vi "test Prepare Aliases for Editor.vi"(8 "error in (no error)":errorcluster, 11 "TestCase in":refnum<class "Routing and Faulting Unit Tests.lvclass">) -> (0 "error out":errorcluster, 3 "TestCase out":refnum<class "Routing and Faulting Unit Tests.lvclass">)   [LabVIEW 2020, in "Routing and Faulting Unit Tests.lvclass"]
uses:
  Routing and Faulting Unit Tests.lvclass
  Shared/Alias Mapping.ctl
  Shared/Alias Endpoint.ctl
  System Explorer/Alias Map by Module.ctl
  System Explorer/Possible Connections.ctl
  Shared/Routing and Faulting Hardware API/Types/Possible Connections for Endpoint.ctl
  <vilib>/addons/_JKI Toolkits/VI Tester/TestCase.llb/TestCase.lvclass
  System Explorer/Routing and Faulting System Explorer.lvlib
  Shared/Routing and Faulting Shared.lvlib
  Shared/Routing and Faulting Hardware API/Routing and Faulting Hardware API.lvlib
  C:/Program Files (x86)/National Instruments/LabVIEW 2020/vi.lib/addons/_JKI Toolkits/VI Tester/TestCase.llb/TestCase.lvclass
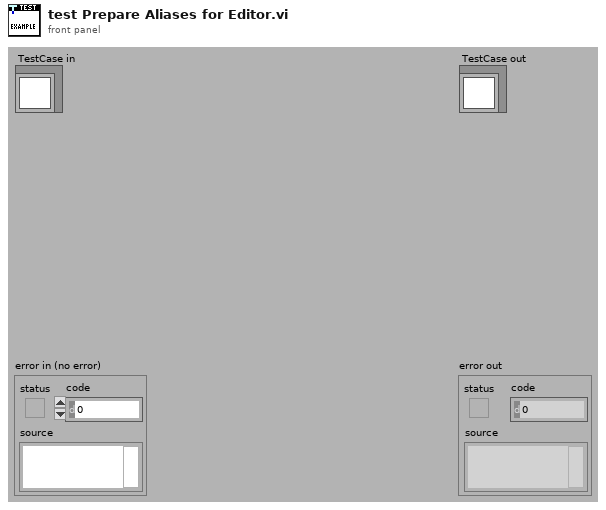
[diagram p1: front panel]
types:
  T1 = typedef "Routing and Faulting System Explorer.lvlib/Possible Connections.ctl" = cluster{" Module Path":string, "Short Module Path":string, "Product Name":string, "Possible Connections":T2[], "Missing":bool}
  T2 = typedef "Routing and Faulting Hardware API.lvlib/Possible Connections for Endpoint.ctl" = cluster{"Source":string, "Destinations":string[]}
  T3 = typedef "Routing and Faulting System Explorer.lvlib/Alias Map by Module.ctl" = cluster{"Module":string, "Alias Map":cluster{"Aliases":string[], "Endpoints":string[]}}
  T4 = typedef "Routing and Faulting Shared.lvlib/Alias Mapping.ctl" = cluster{"Alias":string, "Endpoint":T5}
  T5 = typedef "Routing and Faulting Shared.lvlib/Alias Endpoint.ctl" = cluster{"Module Path":string, "Endpoint":string}
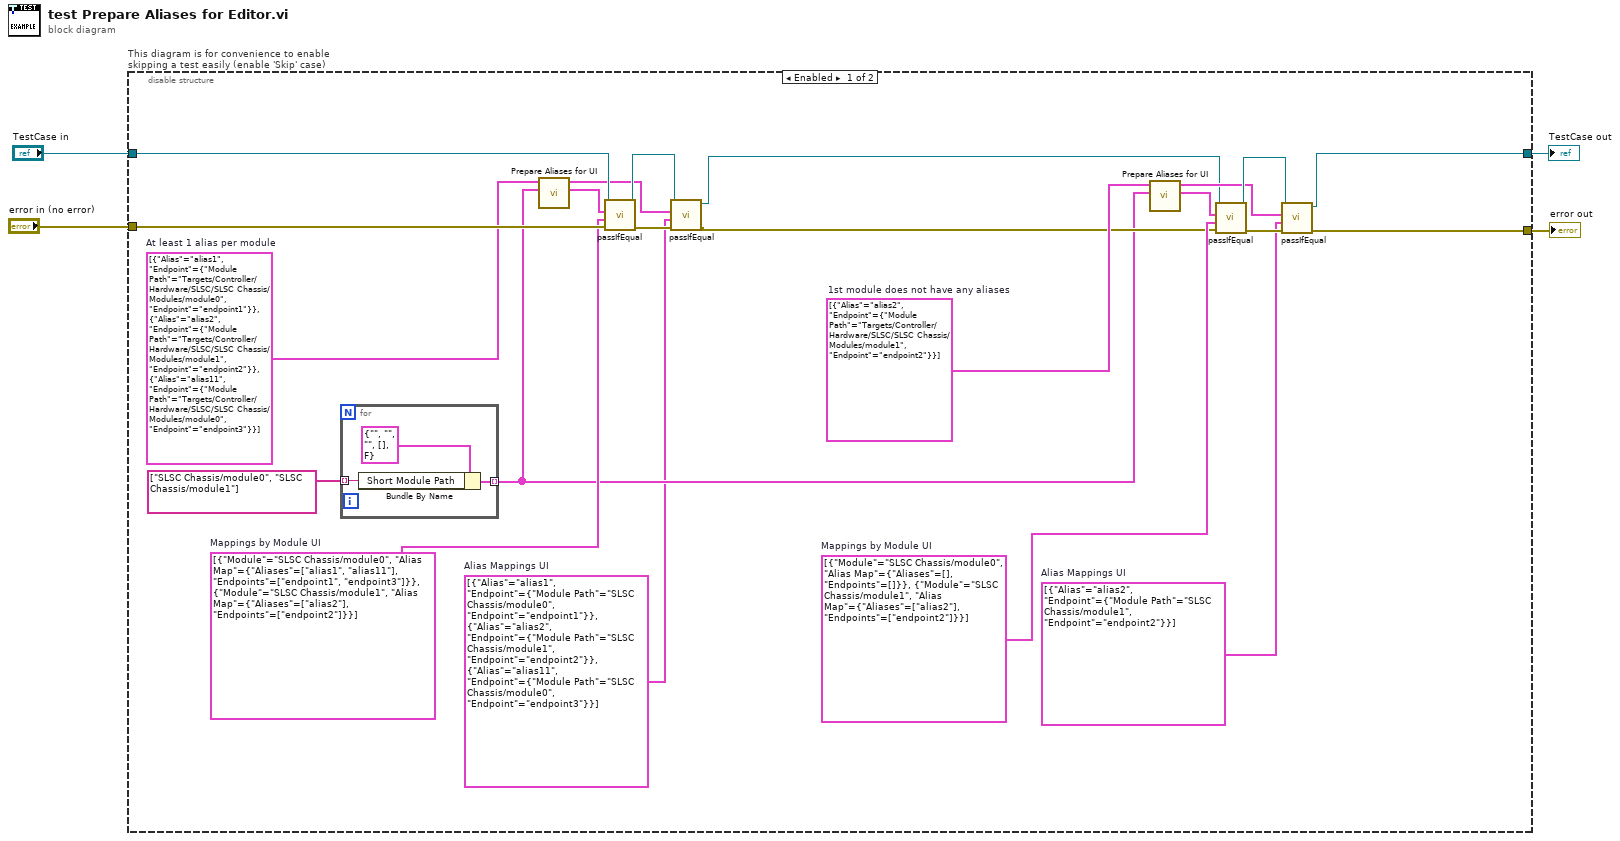
[diagram p0: block diagram]
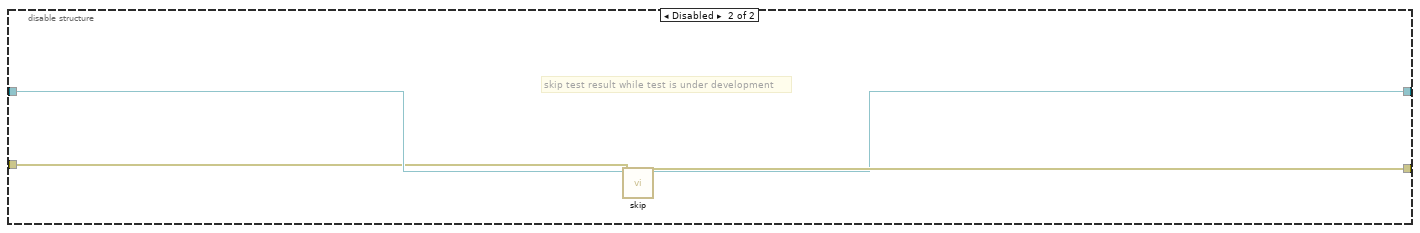
[diagram p2: hidden frame]
diagram:
  n1 = disable-structure "This diagram is for convenience to enable skipping a test easily (enable 'Skip' case)" shown="Enabled" {
    disable-tunnel: "TestCase in" -> [w26 w33]
    disable-tunnel: [w8 w31] -> w1
    disable-tunnel: [w7 w32] -> w3
    disable-tunnel: "error in (no error)" -> [w25 w30]
    frame Enabled {
      w13 = T3[] [{"Module"="SLSC Chassis/module0", "Alias Map"={"Aliases"=[], "Endpoints"=[]}}, {"Module"="SLSC Chassis/module1", "Alias Map"={"Aliases"=["alias2"], "Endpoints"=["endpoint2"]}}]  # Mappings by Module UI
      w11 = T4[] [{"Alias"="alias2", "Endpoint"={"Module Path"="SLSC Chassis/module1", "Endpoint"="endpoint2"}}]  # Alias Mappings UI
      w17 = T4[] [{"Alias"="alias2", "Endpoint"={"Module Path"="Targets/Controller/Hardware/SLSC/SLSC Chassis/Modules/module1", "Endpoint"="endpoint2"}}]  # 1st module does not have any aliases
      w19 = T3[] [{"Module"="SLSC Chassis/module0", "Alias Map"={"Aliases"=["alias1", "alias11"], "Endpoints"=["endpoint1", "endpoint3"]}}, {"Module"="SLSC Chassis/module1", "Alias Map"={"Aliases"=["alias2"], "Endpoints"=["endpoint2"]}}]  # Mappings by Module UI
      w5 = T4[] [{"Alias"="alias1", "Endpoint"={"Module Path"="SLSC Chassis/module0", "Endpoint"="endpoint1"}}, {"Alias"="alias2", "Endpoint"={"Module Path"="SLSC Chassis/module1", "Endpoint"="endpoint2"}}, {"Alias"="alias11", "Endpoint"={"Module Path"="SLSC Chassis/module0", "Endpoint"="endpoint3"}}]  # Alias Mappings UI
      w24 = T4[] [{"Alias"="alias1", "Endpoint"={"Module Path"="Targets/Controller/Hardware/SLSC/SLSC Chassis/Modules/module0", "Endpoint"="endpoint1"}}, {"Alias"="alias2", "Endpoint"={"Module Path"="Targets/Controller/Hardware/SLSC/SLSC Chassis/Modules/module1", "Endpoint"="endpoint2"}}, {"Alias"="alias11", "Endpoint"={"Module Path"="Targets/Controller/Hardware/SLSC/SLSC Chassis/Modules/module0", "Endpoint"="endpoint3"}}]  # At least 1 alias per module
      n2 = for {
        tunnel: string[] ["SLSC Chassis/module0", "SLSC Chassis/module1"] -> [w28] mode=indexing
        tunnel: [w27] -> w6 mode=indexing
        n3 = Bundle By Name(cluster=T1 {" Module Path"="", "Short Module Path"="", "Product Name"="", "Possible Connections"=[], "Missing"=FALSE} ("Item"), "Short Module Path"=w28) -> (w27:T1)
      }
      n4 = call "Prepare Aliases for UI.vi"("Modules and Connections"=w6, "Alias Mappings"=w24) -> ("Mappings by Module UI"=w20:T3[], "Alias Mappings UI"=w18:T4[])  [unwired: 8 in]
      n5 = call-dynamic "passIfEqual.vi"("error in (no error)"=w25, "y"=w19, "x"=w20, "TestCase in"=w26) -> ("error out"=w22:errorcluster, "TestCase out"=w21:refnum<class "Routing and Faulting Unit Tests.lvclass">)  [unwired: 6 in]
      n6 = call-dynamic "passIfEqual.vi"("error in (no error)"=w22, "y"=w5, "x"=w18, "TestCase in"=w21) -> ("error out"=w10:errorcluster, "TestCase out"=w9:refnum<class "Routing and Faulting Unit Tests.lvclass">)  [unwired: 6 in]
      n7 = call "Prepare Aliases for UI.vi"("Modules and Connections"=w6, "Alias Mappings"=w17) -> ("Mappings by Module UI"=w14:T3[], "Alias Mappings UI"=w12:T4[])  [unwired: 8 in]
      n8 = call-dynamic "passIfEqual.vi"("error in (no error)"=w10, "y"=w13, "x"=w14, "TestCase in"=w9) -> ("error out"=w16:errorcluster, "TestCase out"=w15:refnum<class "Routing and Faulting Unit Tests.lvclass">)  [unwired: 6 in]
      n9 = call-dynamic "passIfEqual.vi"("error in (no error)"=w16, "y"=w11, "x"=w12, "TestCase in"=w15) -> ("error out"=w7:errorcluster, "TestCase out"=w8:refnum<class "Routing and Faulting Unit Tests.lvclass">)  [unwired: 6 in]
    }
    frame Disabled {
      # "skip test result while test is under development"
      n10 = call <vilib>:"skip.vi"("error in (no error)"=w30, "TestCase in"=w33) -> ("error out"=w32:errorcluster, "TestCase out"=w31:refnum<class "Routing and Faulting Unit Tests.lvclass">)  [unwired: 8 in]
    }
  }
  "error out" <- w3
  "TestCase out" <- w1
